vi "CreateEvents.vi"(8 "error in (no error)":errorcluster, 11 "JQMHCore in":refnum<class "TemplateModule.lvclass">) -> (0 "error out":errorcluster, 3 "JQMHCore out":refnum<class "TemplateModule.lvclass">)   [LabVIEW 2024, in "TemplateModule.lvclass"]
uses:
  TemplateModule.lvclass
  TemplateModule.lvclass/TemplateModule.ctl
  JQMHCore/Module/RQMHModule.lvclass
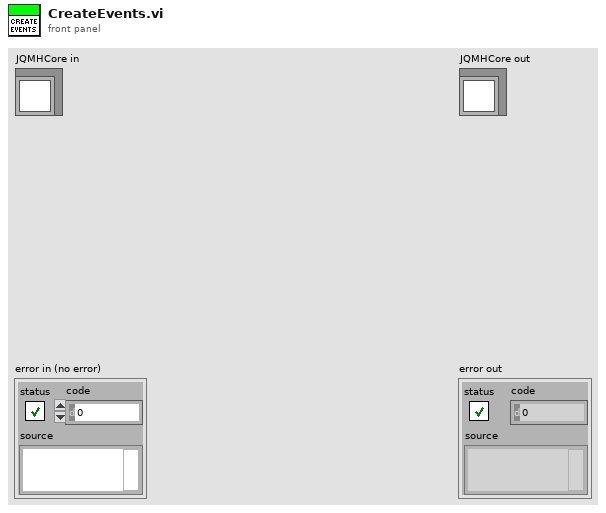
[diagram p1: front panel]
types:
  T1 = typedef "TemplateModule.lvclass/Broadcast Events--cluster.ctl" = cluster{"Stopped":refnum<user-event>, "NewControl258813080":refnum<user-event>, "NewControl260354259":refnum<user-event>}
  T2 = typedef "TemplateModule.lvclass/Request Events--cluster.ctl" = cluster{"Do Something":refnum<user-event>, "NewControl256895198":refnum<user-event>, "NewControl257342523":refnum<user-event>, "NewControl257429121":refnum<user-event>, "NewControl257700474":refnum<user-event>, "NewControl257813921":refnum<user-event>, "NewControl257861065":refnum<user-event>, "NewControl257971046":refnum<user-event>, "NewControl258050239":refnum<user-event>, "NewControl258223653":refnum<user-event>, "NewControl258270105":refnum<user-event>, "NewControl258297343":refnum<user-event>, "NewControl258480234":refnum<user-event>, "NewControl258517903":refnum<user-event>, "NewControl258631628":refnum<user-event>, "NewControl258654618":refnum<user-event>, "NewControl258691941":refnum<user-event>, "NewControl258844085":refnum<user-event>, "NewControl259026866":refnum<user-event>, "NewControl259125042":refnum<user-event>, "NewControl259500026":refnum<user-event>, "NewControl259578961":refnum<user-event>, "NewControl259604365":refnum<user-event>, "NewControl259661713":refnum<user-event>, "NewControl259709857":refnum<user-event>, "NewControl259844037":refnum<user-event>, "NewControl259980850":refnum<user-event>, "NewControl260104585":refnum<user-event>, "NewControl261112600":refnum<user-event>, "NewControl261693191":refnum<user-event>, "NewControl261831553":refnum<user-event>}
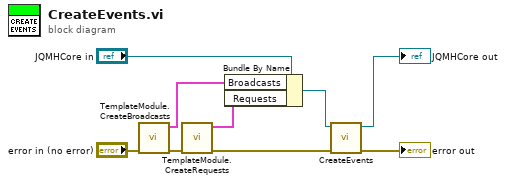
[diagram p0: block diagram]
diagram:
  n1 = call "TemplateModule.CreateBroadcasts.vi"("error in (no error)"="error in (no error)") -> ("error out"=w3:errorcluster, "Broadcasts"=w1:T1)  [unwired: 9 in]
  n2 = call "TemplateModule.CreateRequests.vi"("error in (no error)"=w3) -> ("error out"=w2:errorcluster, "Requests"=w4:T2)  [unwired: 9 in]
  n3 = Bundle By Name(cluster="JQMHCore in", "Broadcasts"=w1, "Requests"=w4) -> (w6:refnum<class "TemplateModule.lvclass">)
  n4 = call-parent "CreateEvents.vi"("error in (no error)"=w2, "JQMHCore in"=w6) -> ("error out"=→"error out":errorcluster, "JQMHCore out"=→"JQMHCore out":refnum<class "TemplateModule.lvclass">)  [unwired: 8 in]
